vi "getData.vi"(8 "error in (no error)":errorcluster, 11 "DeviceData in":refnum<class "DeviceData.lvclass">) -> (0 "error out":errorcluster, 1 "dataArray":dbl[][](array[numeric]), 2 "data out":T1(array[cluster]) {"time" format="%_8g"}, 3 "DeviceData out":refnum<class "DeviceData.lvclass">, 4 "times":dbl[](array[numeric]), 5 "soundStreamPath":path)   [LabVIEW 2009, in "DataMappers.lvlib" / "DeviceData.lvclass"]
uses:
  DeviceData.lvclass
  DatabaseHelpers/Database Objects/Channel/Channel.lvclass
  DeviceData.lvclass/DeviceData.ctl
  SoundDeviceData/SoundDeviceData.lvclass
  DatabaseHelpers/Database Objects/device/device.lvclass
  Scripting/ScriptingEvent/ScriptEventList/ScriptEventList.lvclass
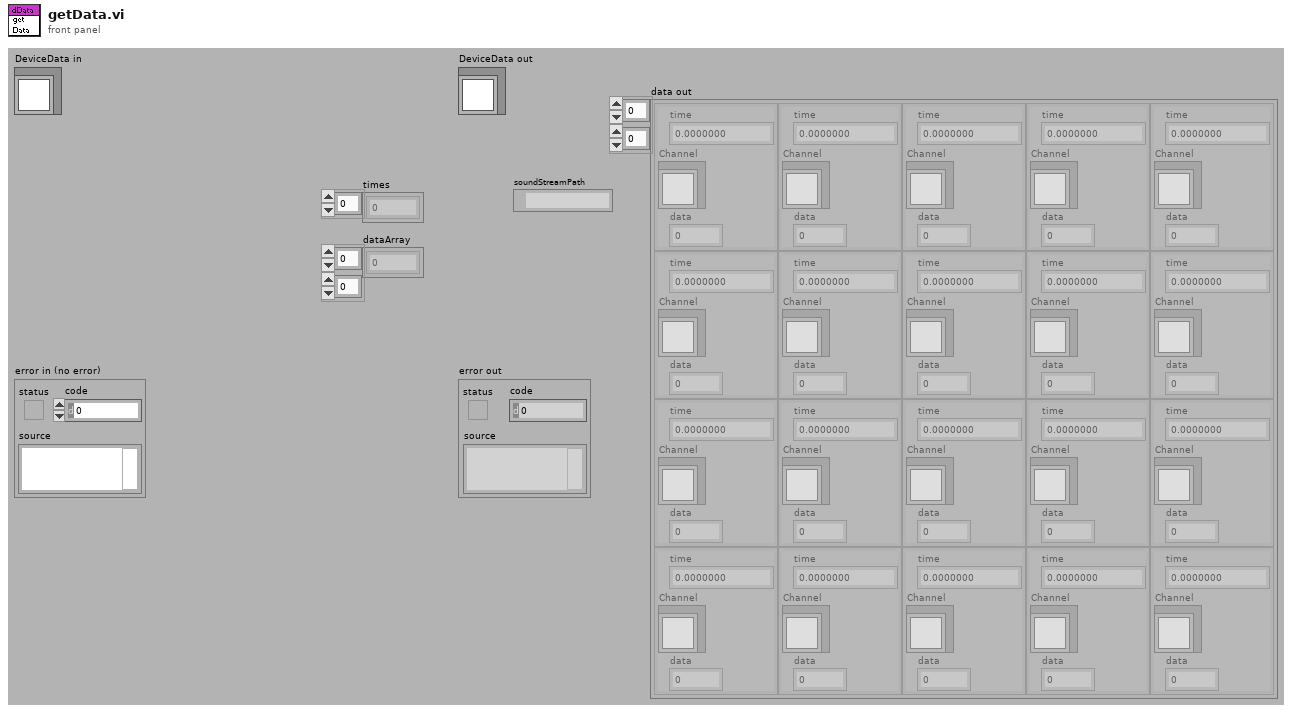
[diagram p1: front panel]
types:
  T1 = cluster{"time":dbl, "Channel":refnum<class "Channel.lvclass">, "data":dbl}[][]
  T2 = cluster{"time":dbl, "Channel":refnum<class "Channel.lvclass">, "value":dbl}[][]
  T3 = cluster{"Channel":refnum<class "Channel.lvclass">, "time":dbl[], "Amplitude":dbl[], "frequency":dbl[], "phase":dbl[]}[]
  T4 = enum16{"eventData", "singleToneData", "fileData"}
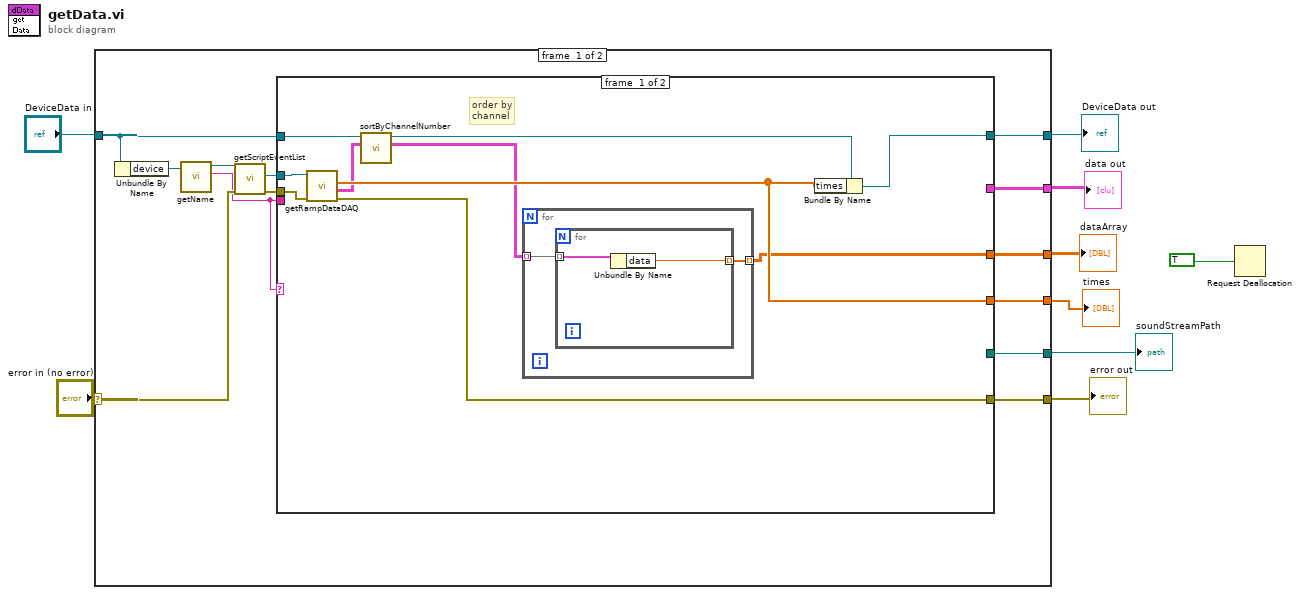
[diagram p0: block diagram]
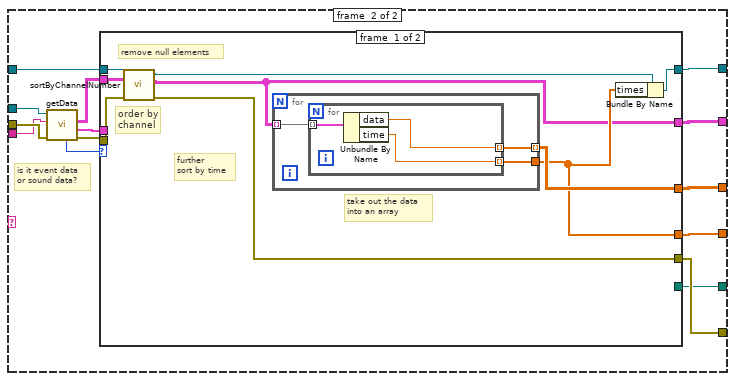
[diagram p2: hidden frame]
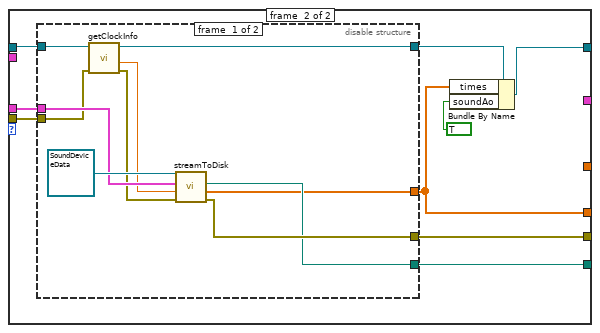
[diagram p3: hidden frame]
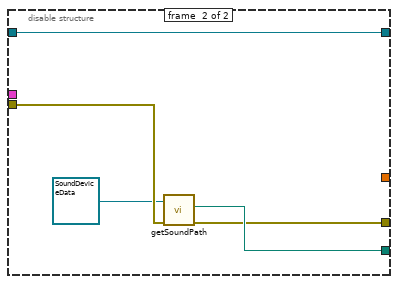
[diagram p4: hidden frame]
diagram:
  n1 = case shown="No Error" "error in (no error)" {
    selector: "error in (no error)" -> [w22 w91]
    tunnel: [w17 w91] -> w8
    tunnel: [w15 w90] -> w6
    tunnel: "DeviceData in" -> [w16 w90]
    tunnel: [w18 _] -> w5
    tunnel: [w19 _] -> w4
    tunnel: [w14 _] -> w3
    tunnel: [w13 _] -> w1
    frame #0 {
      n2 = Unbundle By Name(w16) -> ("device"=w11:refnum<class "device.lvclass">)
      n3 = call "getName.vi"("device.lvclass in"=w11) -> ("name"=w10:string, "device.lvclass out"=w12:refnum<class "device.lvclass">)  [unwired: 8 in, 1 out]
      n4 = call "getScriptEventList.vi"("error in (no error)"=w22, "device.lvclass in"=w12) -> ("error out"=w20:errorcluster, "ScriptEventList"=w21:refnum<class "ScriptEventList.lvclass">)  [unwired: 7 in, 1 out]
      n5 = case shown="Default" w10 {
        tunnel: w21 -> [w32 w50]
        tunnel: w20 -> [w31 w49]
        tunnel: [w23 w48] -> w19
        tunnel: [_ w47] -> w18
        tunnel: [w30 w46] -> w17
        tunnel: w16 -> [w27 w45]
        tunnel: [w28 w42] -> w15
        tunnel: [w29 w41] -> w14
        tunnel: [_ w38] -> w13
        tunnel: w10 -> [_ w37]
        frame #0 {
          # "order by\nchannel"
          n6 = call "getRampDataDAQ.vi"("error in (no error)"=w31, "ScriptEventList in"=w32) -> ("error out"=w30:errorcluster, "data out"=w26:T2, "times out"=w29:dbl[])  [unwired: 6 in, 1 out]
          n7 = call "sortByChannelNumber.vi"("data in"=w26, "DeviceData in"=w27) -> ("data out"=w24:T1, "DeviceData out"=w25:refnum<class "DeviceData.lvclass">)  [unwired: 7 in, 1 out]
          n8 = for {
            tunnel: w24 -> [w34] mode=indexing
            tunnel: [w33] -> w23 mode=indexing
            n9 = for {
              tunnel: w34 -> [w36] mode=indexing
              tunnel: [w35] -> w33 mode=indexing
              n10 = Unbundle By Name(w36) -> ("data"=w35:dbl)
            }
          }
          n11 = Bundle By Name(cluster=w25, "times"=w29) -> (w28:refnum<class "DeviceData.lvclass">)
        }
        frame #1 {
          # "is it event data\nor sound data?"
          n12 = call "getData.vi"("error in (no error)"=w49, "device_name"=w37, "ScriptEventList in"=w50) -> ("error out"=w43:errorcluster, "singleToneData"=w39:T3, "data out"=w44:T1, "dataType"=w40:T4)  [unwired: 4 in, 1 out]
          n13 = case shown="\"singleToneData\"" w40 {
            tunnel: [w59 _] -> w48
            tunnel: [w51 _] -> w47
            tunnel: [w54 w71] -> w46
            tunnel: w45 -> [w55 w68]
            tunnel: w44 -> [w57 _]
            tunnel: w43 -> [w56 w66]
            tunnel: [w53 w74] -> w42
            tunnel: [w58 w69] -> w41
            tunnel: w39 -> [_ w72]
            tunnel: [_ w70] -> w38
            frame #0 {
              # "take out the data\ninto an array"
              # "further\nsort by time"
              # "order by\nchannel"
              # "remove null elements"
              n14 = call "sortByChannelNumber.vi"("error in (no error)"=w56, "data in"=w57, "DeviceData in"=w55) -> ("error out"=w54:errorcluster, "data out"=w51:T1, "DeviceData out"=w52:refnum<class "DeviceData.lvclass">)  [unwired: 6 in]
              n15 = for {
                tunnel: w51 -> [w62] mode=indexing
                tunnel: [w61] -> w59 mode=indexing
                tunnel: [w60] -> w58
                n16 = for {
                  tunnel: w62 -> [w65] mode=indexing
                  tunnel: [w64] -> w61 mode=indexing
                  tunnel: [w63] -> w60 mode=indexing
                  n17 = Unbundle By Name(w65) -> ("data"=w64:dbl, "time"=w63:dbl)
                }
              }
              n18 = Bundle By Name(cluster=w52, "times"=w58) -> (w53:refnum<class "DeviceData.lvclass">)
            }
            frame #1 {
              n19 = disable-structure shown="Enabled" {
                disable-tunnel: w72 -> [w83 _]
                disable-tunnel: [w82 w86] -> w71
                disable-tunnel: [w81 w88] -> w70
                disable-tunnel: [w80 _] -> w69
                disable-tunnel: w68 -> [w79 w89]
                disable-tunnel: [w77 w89] -> w67
                disable-tunnel: w66 -> [w76 w87]
                frame #0 {
                  n20 = call "getClockInfo.vi"("error in (no error)"=w76, "DeviceData in"=w79) -> ("error out"=w75:errorcluster, "masterClockRate"=w78:dbl, "DeviceData out"=w77:refnum<class "DeviceData.lvclass">)  [unwired: 5 in, 2 out]
                  n21 = call "streamToDisk.vi"("error in (no error)"=w75, "sampleRate"=w78, "singleToneData"=w83, "SoundDeviceData in"=refnum<class "SoundDeviceData.lvclass"> refnum ("DataMappers.lvlib:SoundDeviceData.lvclass")) -> ("error out"=w82:errorcluster, "times"=w80:dbl[], "Path"=w81:path)  [unwired: 4 in, 1 out]
                }
                frame #1 {
                  n22 = call "getSoundPath.vi"("error in (no error)"=w87, "SoundDeviceData in"=refnum<class "SoundDeviceData.lvclass"> refnum ("DataMappers.lvlib:SoundDeviceData.lvclass")) -> ("error out"=w86:errorcluster, "Path"=w88:path)  [unwired: 7 in, 1 out]
                }
              }
              n23 = Bundle By Name(cluster=w67, "times"=w69, "soundAo"=TRUE) -> (w74:refnum<class "DeviceData.lvclass">)
            }
          }
        }
      }
    }
    frame #1 {
    }
  }
  "error out" <- w8
  "DeviceData out" <- w6
  "data out" <- w5
  "dataArray" <- w4
  "times" <- w3
  "soundStreamPath" <- w1
  n24 = Request Deallocation(TRUE) -> ()
